vi "Global_Stop.vi"() -> ()   [LabVIEW 2021]
panel:
  in  "stop":bool
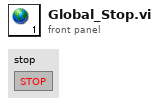
[diagram p1: front panel]
diagram:
